vi "ReturnPathToPublicAppDataControlFile.vi"(8 "error in (no error)":errorcluster) -> (0 "error out":errorcluster, 3 "UIControlsFilePath":path)   [LabVIEW 2019, in "AutoMode.lvlib"]
uses:
  AutoMode.lvlib
  Utilites/Utilities.lvlib
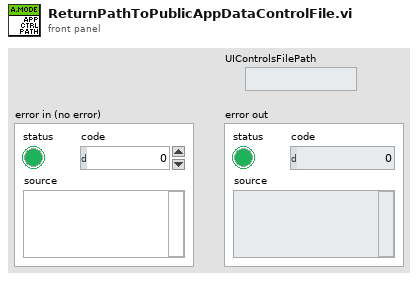
[diagram p1: front panel]
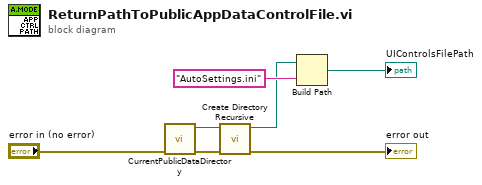
[diagram p0: block diagram]
diagram:
  n1 = call "CurrentPublicDataDirectory.vi"() -> ("Public App Directory"=w3:path)  [unwired: 11 in]
  n2 = call <vilib>:"Create Directory Recursive.vi"("error in (no error)"="error in (no error)", "directory"=w3) -> ("error out"=→"error out":errorcluster, "directory copy"=w4:path)  [unwired: 3 in, 1 out]
  n3 = Build Path(base path=w4, name or relative path="AutoSettings.ini" ("format string")) -> (appended path=→"UIControlsFilePath":path)
